vi "短轴.vi"(8 "y2":dbl, 9 "x2":dbl, 10 "y1":dbl, 11 "x1":dbl) -> (1 "短轴长度":dbl, 2 "第二点y值，x=639":dbl, 3 "第一点y值，x=0":dbl)   [LabVIEW 2015]
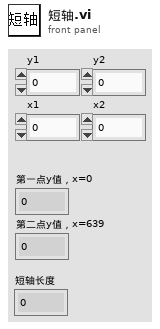
[diagram p1: front panel]
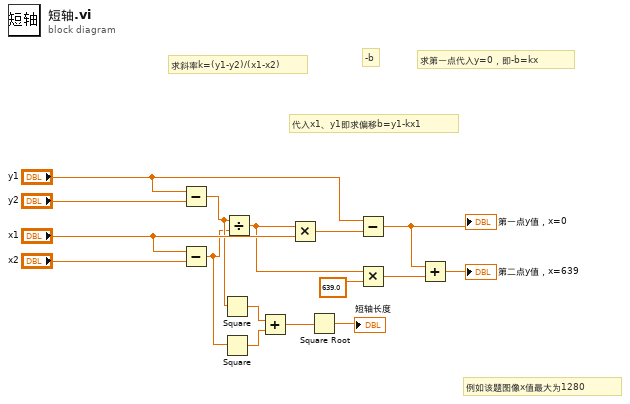
[diagram p0: block diagram]
diagram:
  # "例如该题图像x值最大为1280"
  # "-b"
  # "求第一点代入y=0，即-b=kx"
  # "代入x1、y1即求偏移b=y1-kx1"
  # "求斜率k=(y1-y2)/(x1-x2)"
  n1 = Subtract(x="y1", y="y2") -> (x-y=w6:dbl)
  n2 = Subtract(x="x1", y="x2") -> (x-y=w5:dbl)
  n3 = Square(x=w6) -> (x^2=w4:dbl)
  n4 = Square(x=w5) -> (x^2=w3:dbl)
  n5 = Divide(x=w6, y=w5) -> (x/y=w11:dbl)
  n6 = Add(x=w4, y=w3) -> (x+y=w2:dbl)
  n7 = Multiply(x=w11, y="x1") -> (x*y=w14:dbl)
  n8 = Square Root(x=w2) -> (sqrt(x)=→"短轴长度":dbl)
  n9 = Subtract(x="y1", y=w14) -> (x-y=w8:dbl)
  "第一点y值，x=0" <- w8
  n10 = Multiply(x=w11, y=639.0) -> (x*y=w9:dbl)
  n11 = Add(x=w8, y=w9) -> (x+y=→"第二点y值，x=639":dbl)
